vi "dummy.vi"() -> (3 "standard output":string)   [LabVIEW 2020]
uses:
  serenial.io-ase/ase/ase.lvclass
  common/bin/ase_32-3.dll
panel:
  out "Numeric":i32
  in  "stop":bool
  out "Std Err":string
  out "Std out":string
  out "Remaining StdErr":string
  out "Remaining StdOut":string
  out "ID":string
  out "Exit Code":i32
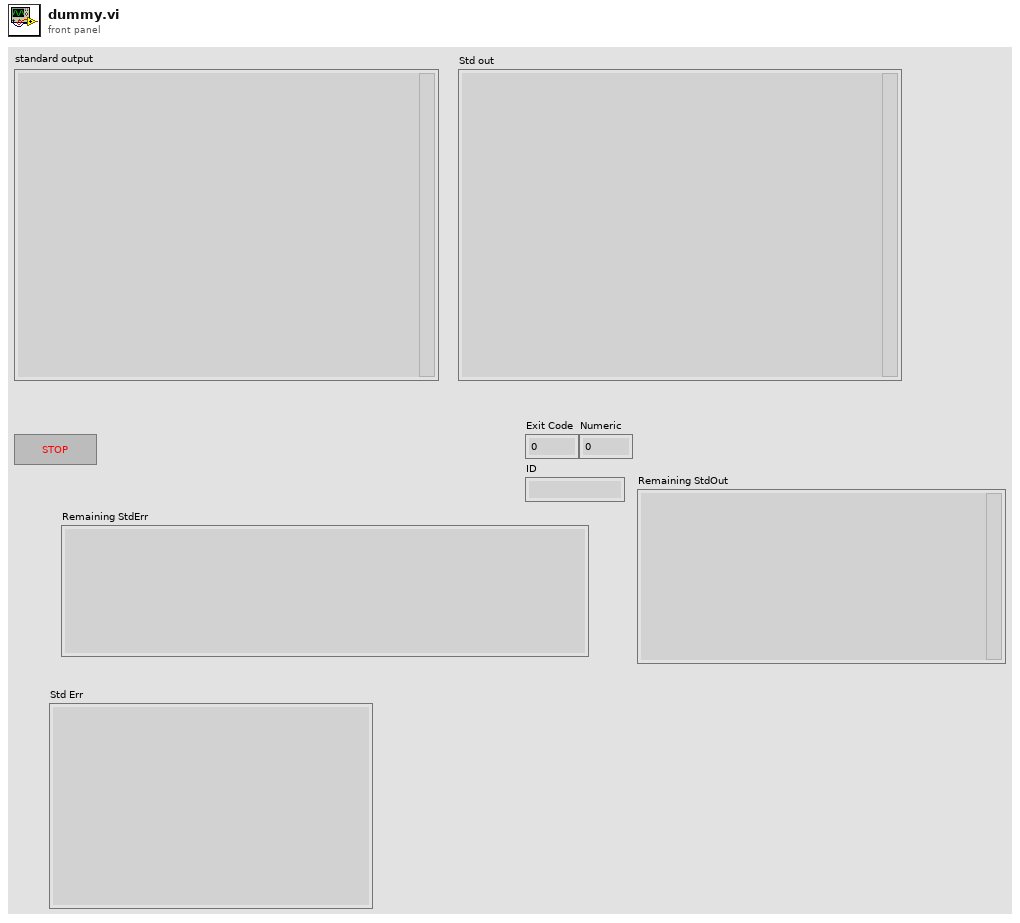
[diagram p1: front panel]
types:
  T1 = typedef "serenial.io-ase.lvlib/ase.lvclass/Event References.ctl" = cluster{"Standard Output":refnum<user-event>, "Standard Error":refnum<user-event>, "Did Exit":refnum<user-event>}
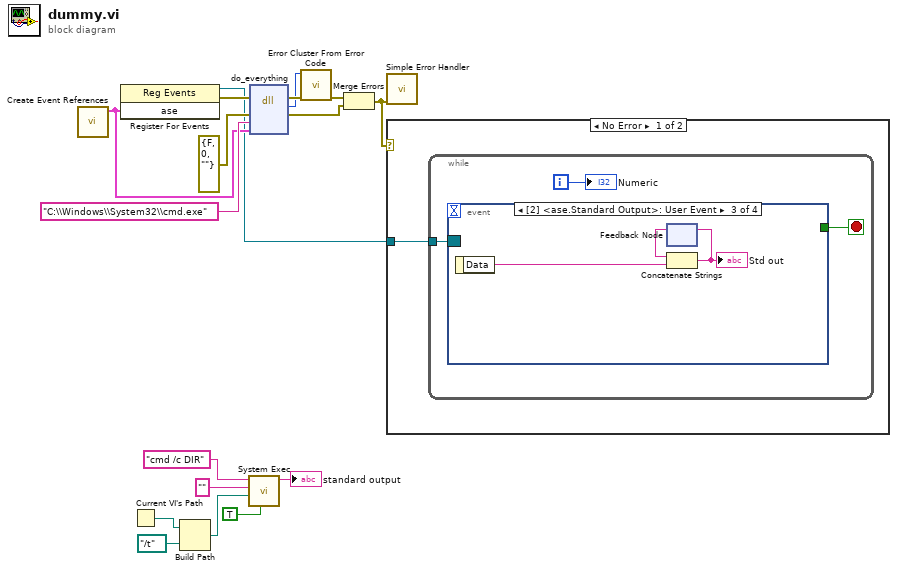
[diagram p0: block diagram]
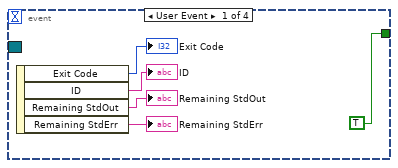
[diagram p2: hidden frame]
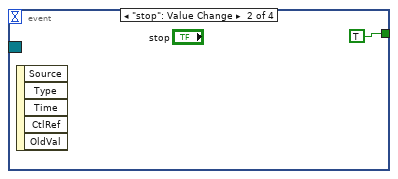
[diagram p3: hidden frame]
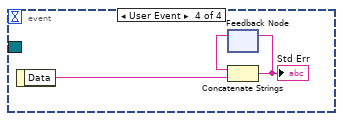
[diagram p4: hidden frame]
diagram:
  n1 = call "Create Event References.vi"() -> ("ase"=w11:T1)  [unwired: 10 in, 1 out]
  n2 = register-events(w11) -> (reference out=w9:refnum<event-registration>, error out=w10:errorcluster)  [unwired: 2 in]
  n3 = Current VI's Path() -> (path=w4:path)
  n4 = Build Path(base path=w4, name or relative path=path "../t") -> (appended path=w7:path)
  n5 = call <vilib>:"System Exec.vi"("run minimized? (F)"=TRUE, "working directory"=w7, "standard input"="", "command line"="cmd /c DIR") -> ("standard output"=→"standard output":string)  [unwired: 4 in, 3 out]
  n6 = dll-call lib="C:/serenial/lib/asynchronous-system-exec/LabVIEW/common/bin/ase_32-3.dll" fn="do_everything"(error in=w10, "error"=errorcluster {"status"=FALSE, "code"=0, "source"=""} ("error constant"), "exe_path"="C:\\Windows\\System32\\cmd.exe", "user_events"=w11) -> (error out=w15:errorcluster, "return type"=w14:i32, "error"=w13:errorcluster)  [unwired: 4 in, 1 out]
  n7 = call <vilib>:"Error Cluster From Error Code.vi"("error in (no error)"=w15, "error code (0)"=w14) -> ("error out"=w16:errorcluster)  [unwired: 7 in]
  n8 = Merge Errors(w16, w13) -> (w8:errorcluster)
  n9 = call <vilib>:"Simple Error Handler.vi"("error in (no error)"=w8) -> ()  [unwired: 4 in, 5 out]
  n10 = case shown="No Error" w8 {
    tunnel: w9 -> [w18 _]
    frame No Error {
      n11 = while {
        tunnel: w18 -> [w21]
        i -> [w19]
        stop <- w20 stop-if-true
        n12 = event shown="[2] <ase.Standard Output>: User Event" {
          selector: w21 -> [_ _ _ _]
          dyn-events: _ -> [_ _ _ _]
          timeout: _ -> [_ _ _ _]
          tunnel: [TRUE TRUE _ _] -> w20
          event User Event {
            n13 = event-data() -> ("Exit Code"=→"Exit Code":i32, "ID"=→"ID":string, "Remaining StdOut"=→"Remaining StdOut":string, "Remaining StdErr"=→"Remaining StdErr":string)  [unwired: 1 in]
          }
          event "stop": Value Change {
            n14 = event-data() -> ()  [unwired: 1 in, 5 out]
          }
          event User Event {
            n15 = event-data() -> ("Data"=w30:string)  [unwired: 1 in]
            n16 = feedback #1() -> (w28:string)  [unwired: 1 in]
            n17 = Concatenate Strings(w28, w30) -> (w29:string)
            "Std out" <- w29
            n18 = feedback-in #1(w29) -> ()
          }
          event User Event {
            n19 = event-data() -> ("Data"=w33:string)  [unwired: 1 in]
            n20 = feedback #2() -> (w31:string)  [unwired: 1 in]
            n21 = Concatenate Strings(w31, w33) -> (w32:string)
            "Std Err" <- w32
            n22 = feedback-in #2(w32) -> ()
          }
        }
        "Numeric" <- w19
      }
    }
    frame Error {
    }
  }
